vi "PCert-Glue-Tree-AddItems.vi"(0 "Tree Ctl Ref":refnum<vi>, 5 "Tree Items to Create":T1[](array[typedef]), 7 "Delete Tree Items First?":bool=TRUE, 9 "Collapse all new items?":bool=TRUE, 11 "error in":errorcluster) -> (4 "Tree Ctl Ref out":refnum<vi>, 6 "Tree Item Tags Created":string[](array[string]), 15 "error out":errorcluster)   [LabVIEW 2013]
uses:
  PCert-Glue-TreeItem.ctl
panel:
  # "Inputs"
  # "Outputs"
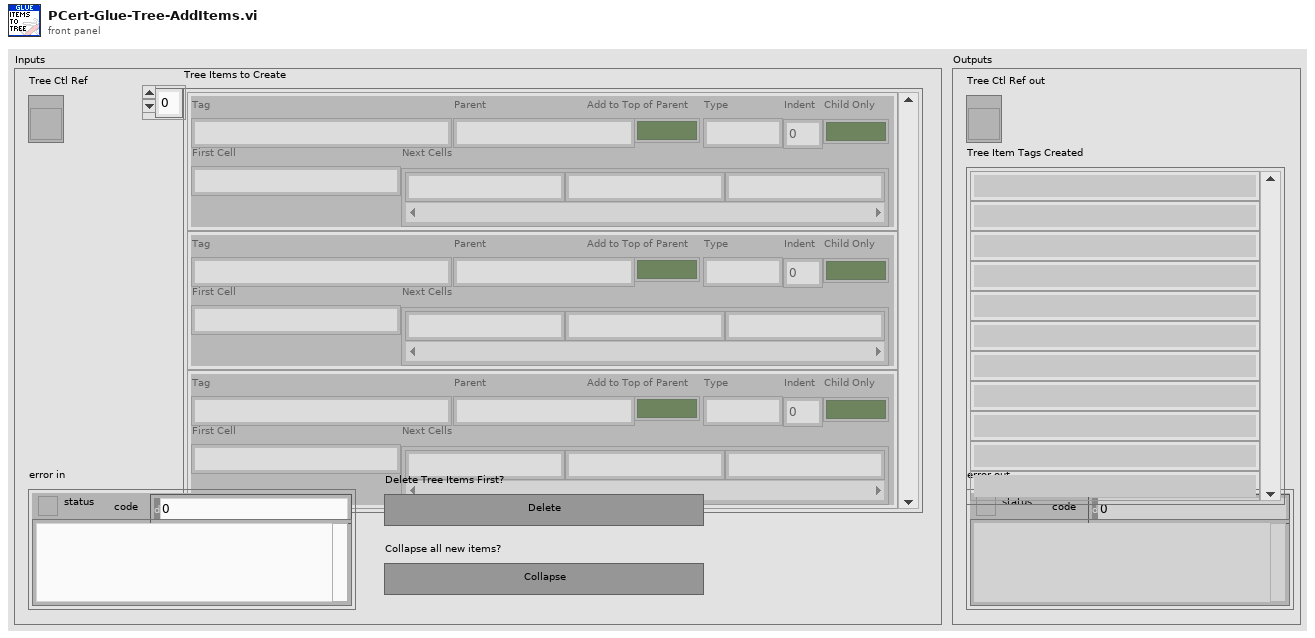
[diagram p1: front panel]
types:
  T1 = typedef "PCert-Glue-TreeItem.ctl" = cluster{"Tag":string, "Parent":string, "Add to Top of Parent":bool, "Type":string, "Indent":i32, "Child Only":bool, "First Cell":string, "Next Cells":string[]}
  T2 = cluster{"Left Cell String":string, "Child Text":string[], "Child Tag":string, "Item Indent":i32, "Child Only?":bool, "Glyph Index":i32}
  T3 = cluster{"Position":i32, "Tag":string, "Parent":string}
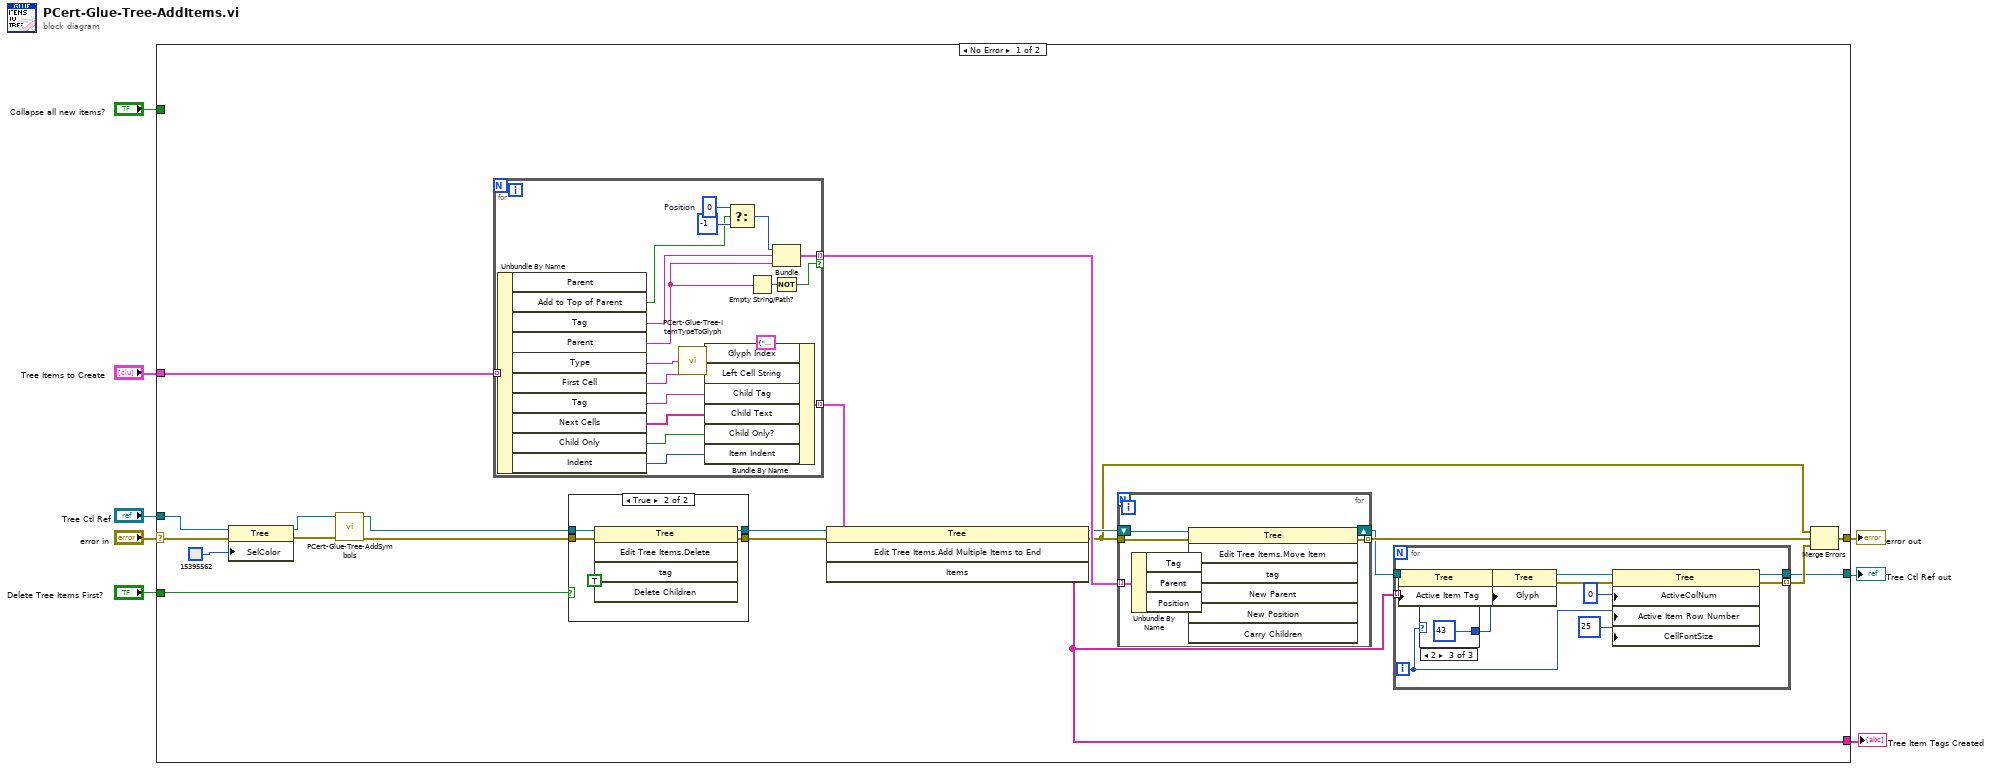
[diagram p0: block diagram]
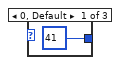
[diagram p2: hidden frame]
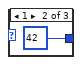
[diagram p3: hidden frame]
diagram:
  n1 = case shown="No Error" "error in" {
    selector: "error in" -> [w13 w80]
    tunnel: [w26 w80] -> w8
    tunnel: "Tree Ctl Ref" -> [w12 w79]
    tunnel: "Tree Items to Create" -> [w27 _]
    tunnel: "Delete Tree Items First?" -> [w23 _]
    tunnel: "Collapse all new items?" -> [_ _]
    tunnel: [w19 _] -> w2
    tunnel: [w14 w79] -> w1
    frame No Error {
      n2 = property class="Tree"(reference=w12, error in=w13, "SelColor"=u32 15395562) -> (reference out=w10:refnum<vi>, error out=w11:errorcluster)
      n3 = call "PCert-Glue-Tree-AddSymbols.vi"("error in (no error)"=w11, "TreeControl in"=w10) -> ("error out"=w20:errorcluster, "TreeControl out"=w21:refnum<vi>)  [unwired: 8 in]
      n4 = for {
        tunnel: [w69] -> w29 mode=indexing
        tunnel: w27 -> [w70] mode=indexing
        tunnel: [w52] -> w28 mode=indexing if=w57
        w59 = 0  # Position
        n5 = Unbundle By Name(w70) -> ("Add to Top of Parent"=w56:bool, "Tag"=w53:string, "Parent"=w54:string, "Type"=w68:string, "First Cell"=w67:string, "Tag"=w65:string, "Next Cells"=w64:string[], "Child Only"=w63:bool, "Indent"=w62:i32)  [unwired: 1 out]
        n6 = call "PCert-Glue-Tree-ItemTypeToGlyph.vi"("Item Type"=w68) -> ("Glyph Index"=w66:i32)  [unwired: 1 in, 2 out]
        n7 = Bundle By Name(cluster=T2 {"Left Cell String"="", "Child Text"=[], "Child Tag"="", "Item Indent"=0, "Child Only?"=FALSE, "Glyph Index"=0} ("Item"), "Glyph Index"=w66, "Left Cell String"=w67, "Child Tag"=w65, "Child Text"=w64, "Child Only?"=w63, "Item Indent"=w62) -> (w69:T2)
        n8 = Select(t=w59, s=w56, f=-1) -> (s? t:f=w55:i32)
        n9 = Empty String/Path?(string/path=w54) -> (empty?=w61:bool)
        n10 = Bundle("Position"=w55, "Tag"=w53, "Parent"=w54) -> (w52:T3)  [unwired: 1 in]
        n11 = Not(x=w61) -> (.not. x?=w57:bool)
      }
      n12 = case shown="True" w23 {
        tunnel: w21 -> [w46 w50]
        tunnel: [w46 w49] -> w18
        tunnel: w20 -> [w45 w48]
        tunnel: [w45 w47] -> w24
        frame False {
        }
        frame True {
          n13 = invoke on="Invoke Node" class="Tree" method="Edit Tree Items.Delete"(reference=w50, error in=w48, "Delete Children"=TRUE ("Delete Children?")) -> (reference out=w49:refnum<vi>, error out=w47:errorcluster)  [unwired: 2 in, 3 out]
        }
      }
      n14 = invoke on="Invoke Node" class="Tree" method="Edit Tree Items.Add Multiple Items to End"(reference=w18, error in=w24, "Items"=w29) -> (reference out=w25:refnum<vi>, error out=w15:errorcluster, "Edit Tree Items:Add Multiple Items to End"=w19:string[])  [unwired: 1 in, 1 out]
      n15 = for {
        tunnel: w15 -> [w78]
        tunnel: [w77] -> w22 mode=indexing
        tunnel: w28 -> [w75] mode=indexing
        shift-right: [w71] -> w17
        shift-left: w25 -> [w76]
        n16 = Unbundle By Name(w75) -> ("Tag"=w74:string, "Parent"=w73:string, "Position"=w72:i32)
        n17 = invoke on="Invoke Node" class="Tree" method="Edit Tree Items.Move Item"(reference=w76, error in=w78, "tag"=w74, "New Parent"=w73, "New Position"=w72) -> (reference out=w71:refnum<vi>, error out=w77:errorcluster)  [unwired: 2 in, 5 out]
      }
      n18 = for {
        tunnel: w19 -> [w38] mode=indexing
        tunnel: w17 -> [w37]
        tunnel: [w31] -> w16 mode=indexing
        tunnel: [w30] -> w14
        i -> [w32]
        n19 = property class="Tree"(reference=w37, "Active Item Tag"=w38) -> (reference out=w41:refnum<vi>, error out=w40:errorcluster)  [unwired: 1 in]
        n20 = case shown="2" w32 {
          tunnel: [41 ("Active Item:Symbol Index") 42 ("Active Item:Symbol Index") 43 ("Active Item:Symbol Index")] -> w39
          frame 0, Default {
          }
          frame 1 {
          }
          frame 2 {
          }
        }
        n21 = property class="Tree"(reference=w41, error in=w40, "Glyph"=w39) -> (reference out=w33:refnum<vi>, error out=w34:errorcluster)
        n22 = property class="Tree"(reference=w33, error in=w34, "ActiveColNum"=0 ("Active Cell:Active Column Number"), "Active Item Row Number"=w32, "CellFontSize"=u32 25 ("Active Cell:Cell Font:Size")) -> (reference out=w30:refnum<vi>, error out=w31:errorcluster)
      }
      n23 = Merge Errors(w15, w22, w16) -> (w26:errorcluster)
    }
    frame Error {
    }
  }
  "error out" <- w8
  "Tree Ctl Ref out" <- w1
  "Tree Item Tags Created" <- w2
